vi "Set Formatter.vi"(10 "formatter":refnum<class "Formatter.lvclass">, 11 "handler in":refnum<class "Formatting Handler.lvclass">) -> (3 "handler out":refnum<class "Formatting Handler.lvclass">)   [LabVIEW 2018, in "GLog.lvlib" / "Formatting Handler.lvclass"]
uses:
  Formatting Handler.lvclass
  formatter_interface/Formatter.lvclass
  Formatting Handler.lvclass/Formatting Handler.ctl
panel:
  # "Connector Pane"
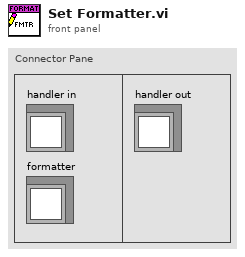
[diagram p1: front panel]
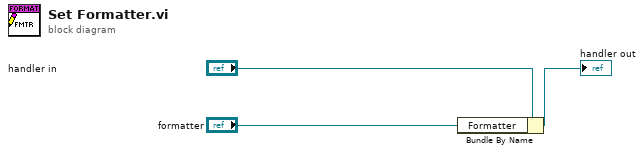
[diagram p0: block diagram]
diagram:
  n1 = Bundle By Name(cluster="handler in", "Formatter"="formatter") -> (→"handler out":refnum<class "Formatting Handler.lvclass">)
